vi "Antrenare_Retea.vi"() -> ()   [LabVIEW 2024]
uses:
  <vilib>/National Instruments/NI Super Simple Neural Networks/API/Create 1 Hidden Layer.vi
  <vilib>/Utility/file.llb/Read Delimited Spreadsheet (DBL).vi
  <vilib>/National Instruments/NI Super Simple Neural Networks/Neural Network.lvclass
panel:
  in  "Meteo Data Input":path
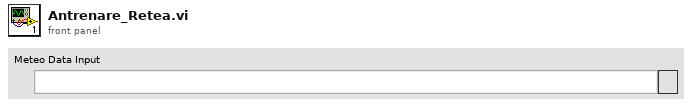
[diagram p1: front panel]
types:
  T1 = enum16{"open", "replace", "create", "open or create", "replace or create", "replace or create with confirmation"}
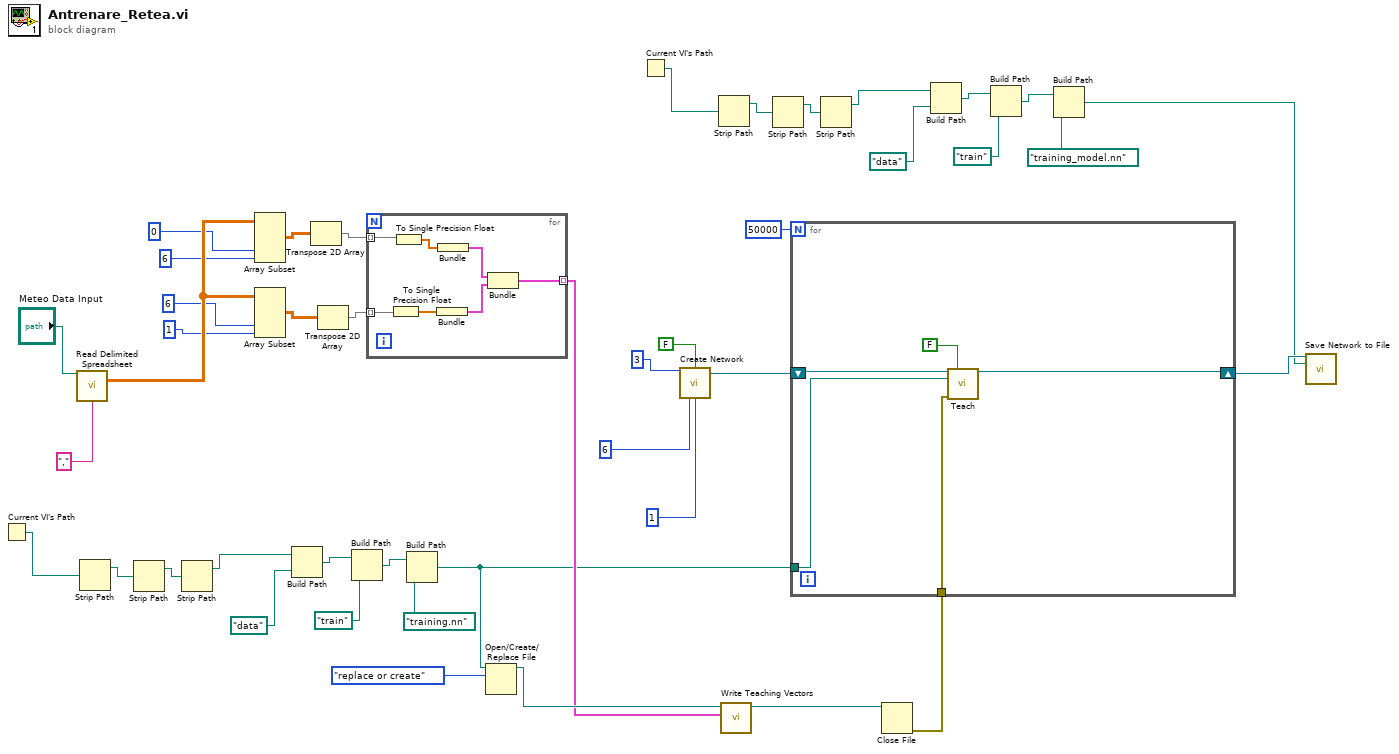
[diagram p0: block diagram]
diagram:
  n1 = Current VI's Path() -> (path=w20:path)
  n2 = call-poly <vilib>:"Read Delimited Spreadsheet.vi"("file path (dialog if empty)"="Meteo Data Input", "delimiter (\\t)"="," ("delimiter (\\t)")) -> ("all rows"=w35:dbl[][])  [unwired: 8 in, 5 out]
  n3 = Strip Path(path=w20) -> (stripped path=w19:path)  [unwired: 1 out]
  n4 = Strip Path(path=w19) -> (stripped path=w18:path)  [unwired: 1 out]
  n5 = Strip Path(path=w18) -> (stripped path=w12:path)  [unwired: 1 out]
  n6 = Array Subset(array=w35, index (col)=0 ("index"), length (col)=6 ("length")) -> (w25:dbl[][])  [unwired: 2 in]
  n7 = Array Subset(array=w35, index (col)=6 ("index"), length (col)=1 ("length")) -> (w23:dbl[][])  [unwired: 2 in]
  n8 = Build Path(base path=w12, name or relative path=path "data") -> (appended path=w17:path)
  n9 = Transpose 2D Array(2D array=w25) -> (transposed array=w24:dbl[][])
  n10 = Transpose 2D Array(2D array=w23) -> (transposed array=w22:dbl[][])
  n11 = Build Path(base path=w17, name or relative path=path "train") -> (appended path=w16:path)
  n12 = for {
    tunnel: w22 -> [w50] mode=indexing
    tunnel: w24 -> [w49] mode=indexing
    tunnel: [w44] -> w34 mode=indexing
    n13 = To Single Precision Float(number=w50) -> (single precision float=w47:sgl[])
    n14 = To Single Precision Float(number=w49) -> (single precision float=w48:sgl[])
    n15 = Bundle(w47) -> (w45:cluster{sgl[]})  [unwired: 1 in]
    n16 = Bundle(w48) -> (w46:cluster{sgl[]})  [unwired: 1 in]
    n17 = Bundle(w46, w45) -> (w44:cluster{cluster{sgl[]}, cluster{sgl[]}})  [unwired: 1 in]
  }
  n18 = Build Path(base path=w16, name or relative path=path "training.nn") -> (appended path=w11:path)
  n19 = Open/Create/Replace File(file path (use dialog)=w11, operation (0:open)=T1."replace or create") -> (refnum out=w36:refnum<file>)  [unwired: 4 in, 2 out]
  n20 = Current VI's Path() -> (path=w10:path)
  n21 = call-poly <vilib>:"Create Network.vi"("1st Hidden Layer Neurons"=u32 3 ("2nd Hidden Layer Neurons"), "Add Bias Inputs (True)"=FALSE, "# Inputs"=6 ("length"), "Output Neurons/Outputs"=u32 1) -> ("Neural Network Out"=w40:refnum<class "Neural Network.lvclass">)  [unwired: 10 in, 1 out]
  n22 = Strip Path(path=w10) -> (stripped path=w9:path)  [unwired: 1 out]
  n23 = call <vilib>:"Write Teaching Vectors.vi"("Teaching Vectors"=w34, "Teaching File Ref In"=w36) -> ("Teaching File Ref Out"=w33:refnum<file>)  [unwired: 8 in, 1 out]
  n24 = Strip Path(path=w9) -> (stripped path=w8:path)  [unwired: 1 out]
  n25 = Strip Path(path=w8) -> (stripped path=w3:path)  [unwired: 1 out]
  n26 = Close File(refnum=w33) -> (error out=w32:errorcluster)  [unwired: 1 in, 1 out]
  n27 = for {
    N: 50000 -> [_]
    shift-right: [w52] -> w31
    shift-left: w40 -> [w55]
    tunnel: w32 -> [w54]
    tunnel: w11 -> [w51]
    n28 = call <vilib>:"Teach.vi"("Neural Network In"=w55, "Enable Growing/Prunning"=FALSE, "Teaching Set Path In"=w51, "Error In"=w54) -> ("Neural Network Out"=w52:refnum<class "Neural Network.lvclass">)  [unwired: 7 in, 4 out]
  }
  n29 = Build Path(base path=w3, name or relative path=path "data") -> (appended path=w7:path)
  n30 = Build Path(base path=w7, name or relative path=path "train") -> (appended path=w6:path)
  n31 = Build Path(base path=w6, name or relative path=path "training_model.nn") -> (appended path=w1:path)
  n32 = call <vilib>:"Save Network to File.vi"("Neural Network In"=w31, "File Path (dialog)"=w1) -> ()  [unwired: 11 in, 3 out]
